vi "Stop Core.vi"(10 "final error code":i32, 11 "Nested in":refnum<class "Root.lvclass">) -> (3 "Nested out":refnum<class "Root.lvclass">)   [LabVIEW 2025, in "Root.lvlib" / "Root.lvclass"]
doc: "(<B>Filename</B>: Actor Framework.lvlib:Actor.lvclass:Stop Core.vi)\n\nDefines what the actor does before it stops. Use the <B>final error code</B> input to determine whether the actor shut down in response to an error.\n\nBy default, this method does nothing. A descendant class may override it to define behavior, such as shutting down any processes the actor initiated in its override of the Actor Core method."
uses:
  Root.lvclass
  Root.lvclass/Root.ctl
  <vilib>/ActorFramework/Actor/Actor.lvclass
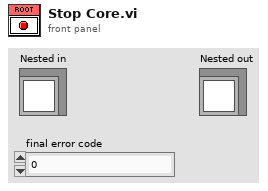
[diagram p1: front panel]
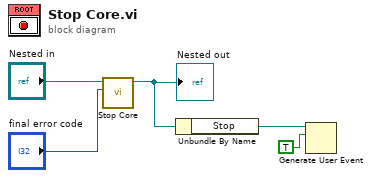
[diagram p0: block diagram]
diagram:
  n1 = call-parent "Stop Core.vi"("final error code"="final error code", "Actor in"="Nested in") -> ("Actor out"=w3:refnum<class "Root.lvclass">)  [unwired: 9 in]
  "Nested out" <- w3
  n2 = Unbundle By Name(w3) -> ("Stop"=w1:refnum<user-event>)
  n3 = Generate User Event(user event=w1, event data cluster=TRUE ("event data")) -> ()  [unwired: 2 in, 2 out]
